vi "main.vi"() -> ()   [LabVIEW 2023]
panel:
  out "6-5 2":string
  out "6-4 2":string
  out "6-3 2":string
  out "6-2 2":string
  out "6-1 2":string
  out "5-5 2":string
  out "5-4 2":string
  out "5-3 2":string
  out "5-2 2":string
  out "5-1 2":string
  out "4-5 2":string
  out "4-4 2":string
  out "4-3 2":string
  out "4-2 2":string
  out "4-1 2":string
  out "3-5 2":string
  out "3-4 2":string
  out "3-3 2":string
  out "3-2 2":string
  out "3-1 2":string
  out "2-5 2":string
  out "2-4 2":string
  out "2-3 2":string
  out "2-2 2":string
  out "2-1 2":string
  out "1-5 2":string
  out "1-4 2":string
  out "1-3 2":string
  out "1-2 2":string
  out "1-1 2":string
  out "Class Name":string
  out "row":i32
  out "column":i32
  in  "BACKSPACE":bool
  in  "M":bool
  in  "N":bool
  in  "B":bool
  in  "V":bool
  in  "C":bool
  in  "X":bool
  in  "Z":bool
  in  "ENTER":bool
  in  "L":bool
  in  "K":bool
  in  "J":bool
  in  "H":bool
  in  "G":bool
  in  "F":bool
  in  "D":bool
  in  "S":bool
  in  "A":bool
  in  "P":bool
  in  "O":bool
  in  "I":bool
  in  "U":bool
  in  "Y":bool
  in  "T":bool
  in  "R":bool
  in  "E":bool
  in  "W":bool
  in  "Q":bool
  out "6-5":string
  out "6-4":string
  out "6-3":string
  out "6-2":string
  out "6-1":string
  out "5-5":string
  out "5-4":string
  out "5-3":string
  out "5-2":string
  out "5-1":string
  out "4-5":string
  out "4-4":string
  out "4-3":string
  out "4-2":string
  out "4-1":string
  out "3-5":string
  out "3-4":string
  out "3-3":string
  out "3-2":string
  out "3-1":string
  out "2-5":string
  out "2-4":string
  out "2-3":string
  out "2-2":string
  out "2-1":string
  out "1-5":string
  out "1-4":string
  out "1-3":string
  out "1-2":string
  out "1-1":string
  out "Array 2":string[](array[string])
  out "Array 3":string[][](array[string])
  # "Wordle"
  # "Wordle AI"
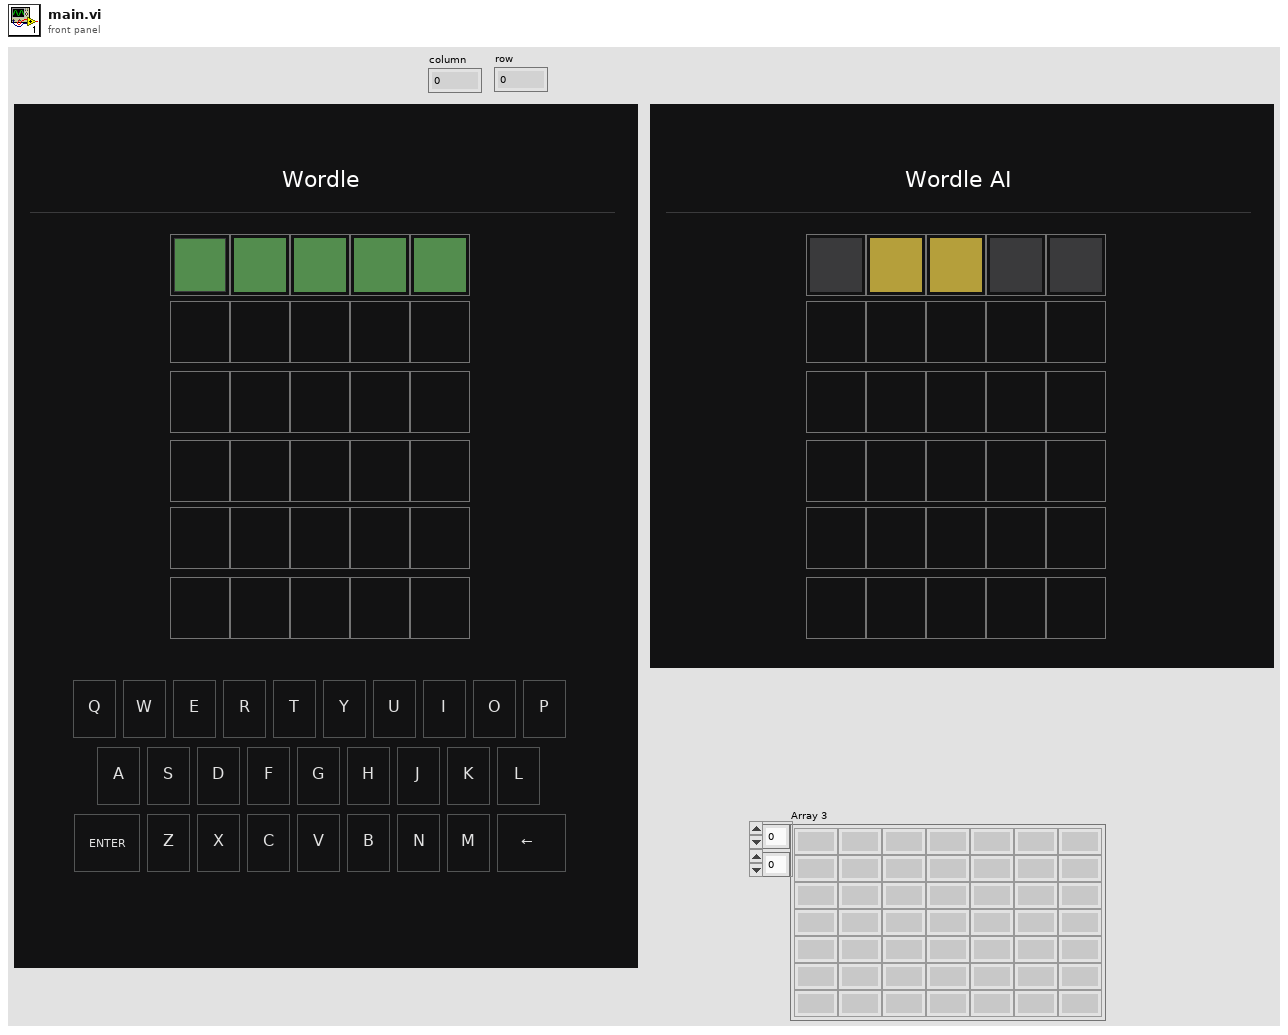
[diagram p1: front panel]
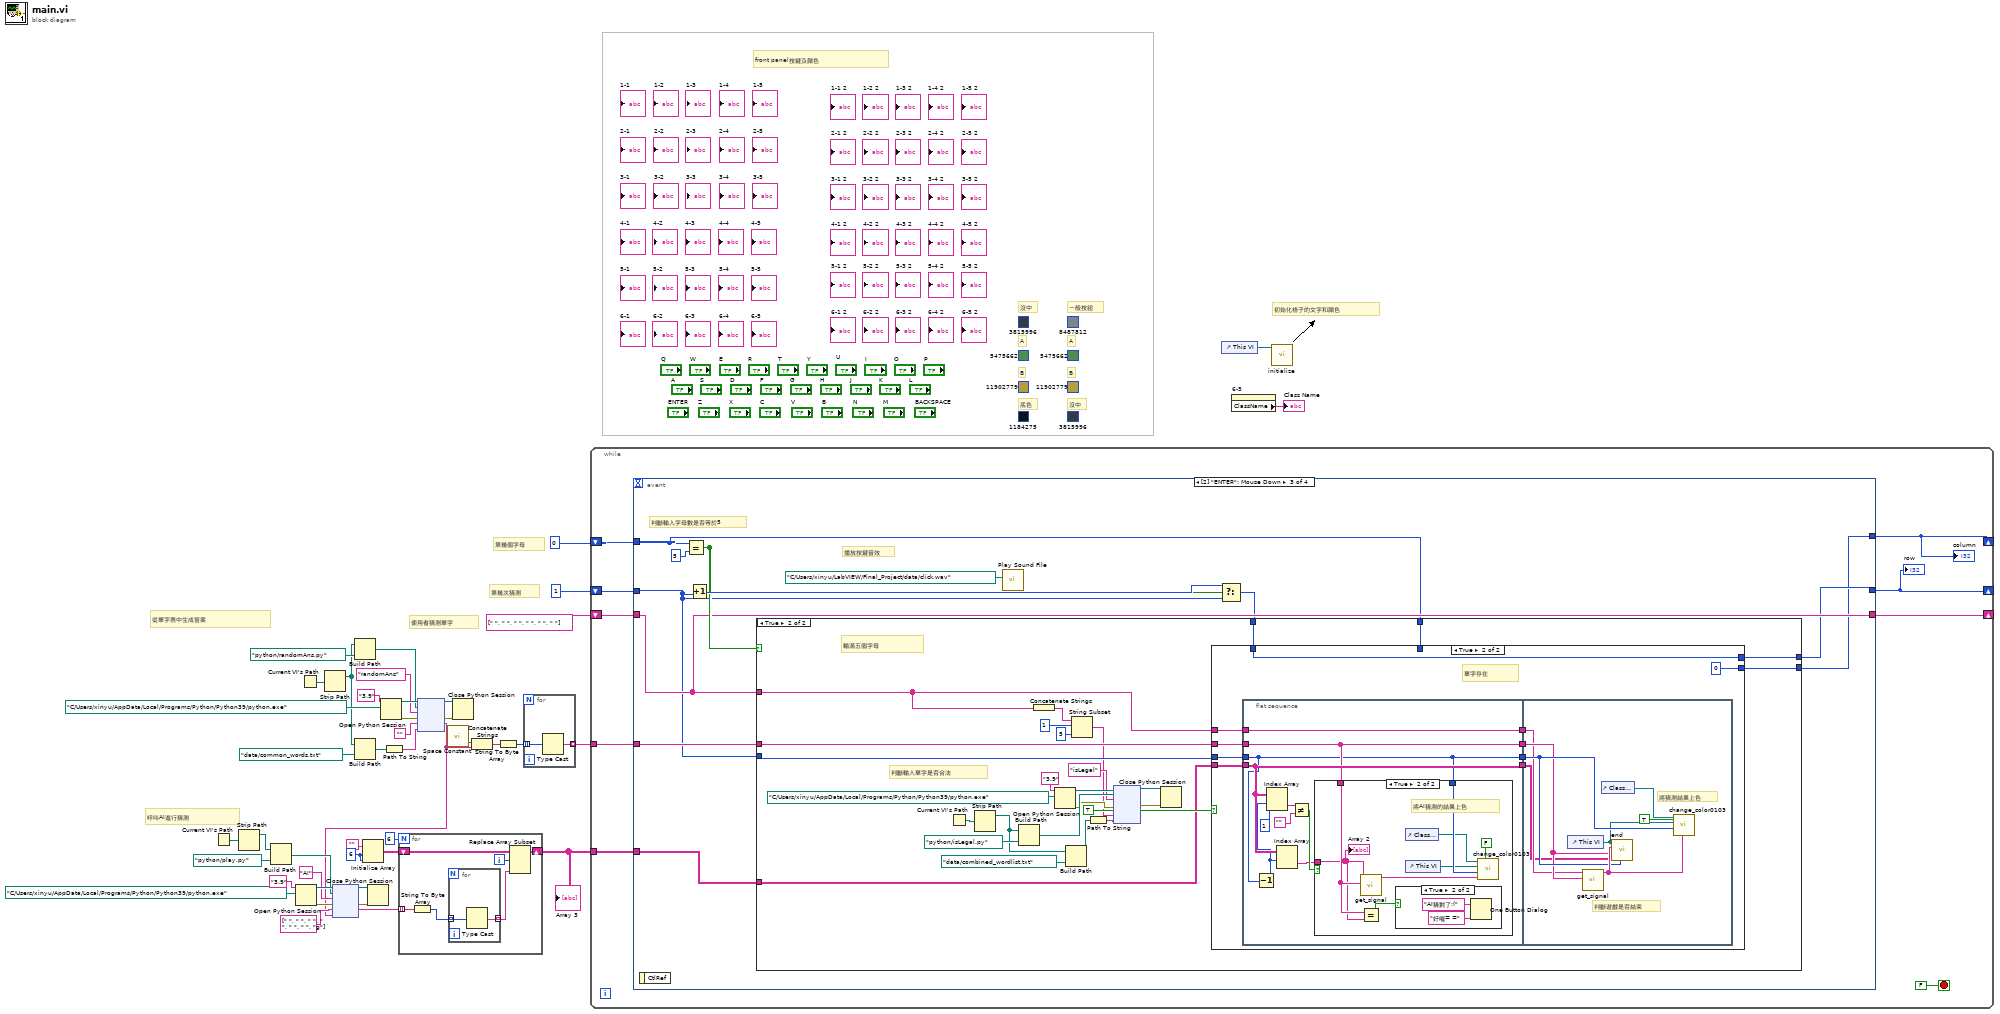
[diagram p0: block diagram]
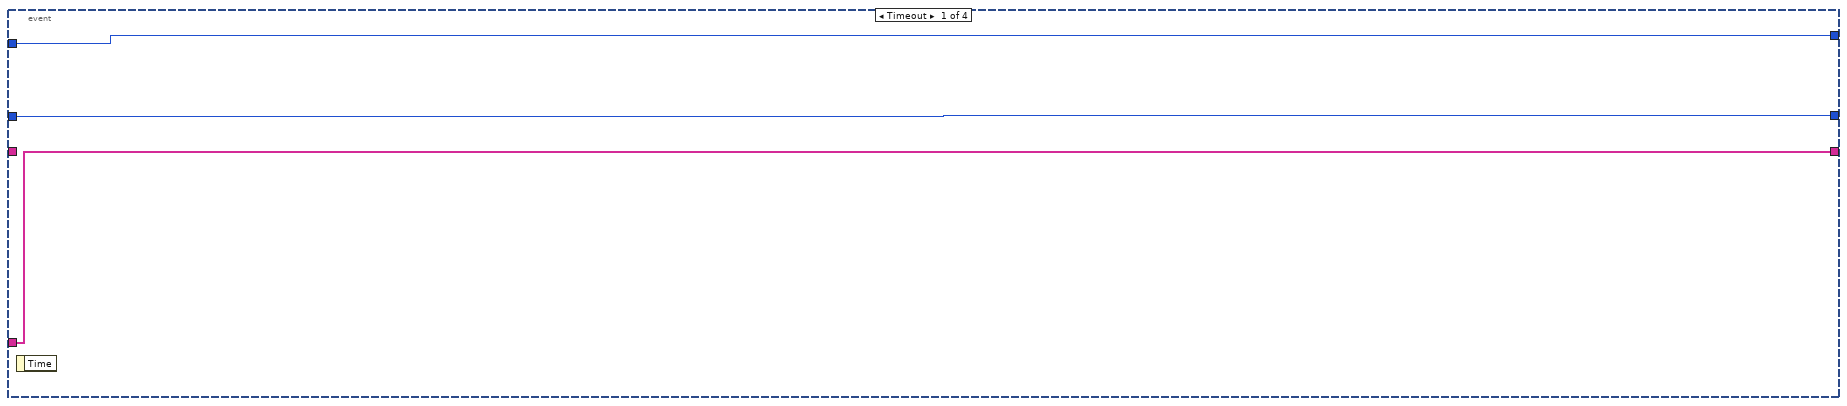
[diagram p2: hidden frame]
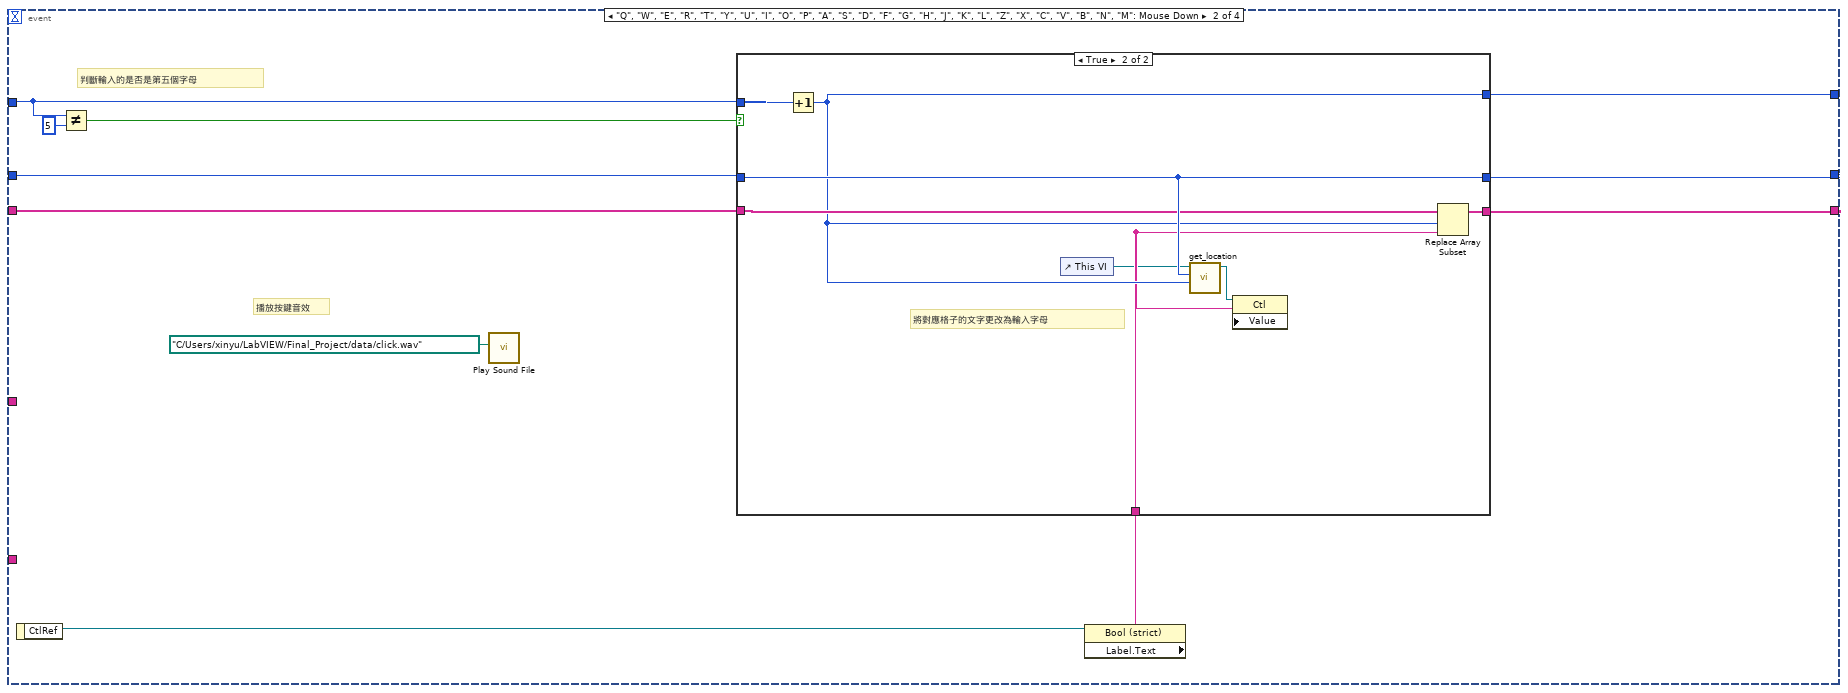
[diagram p3: hidden frame]
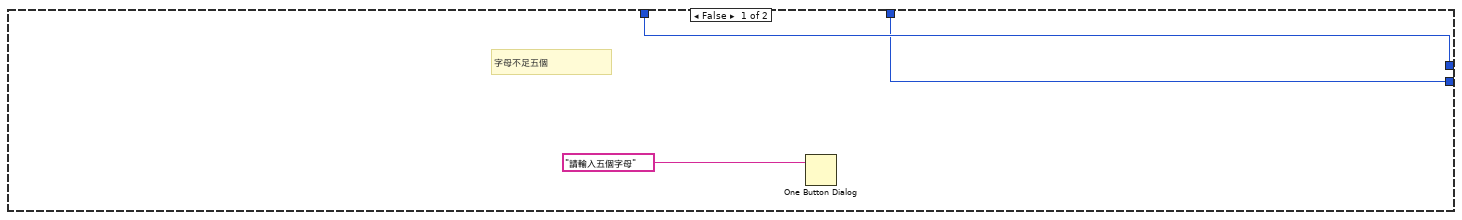
[diagram p5: hidden frame]
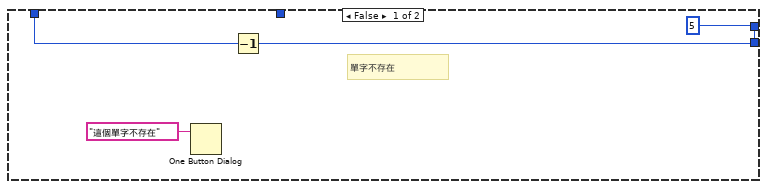
[diagram p6: hidden frame]
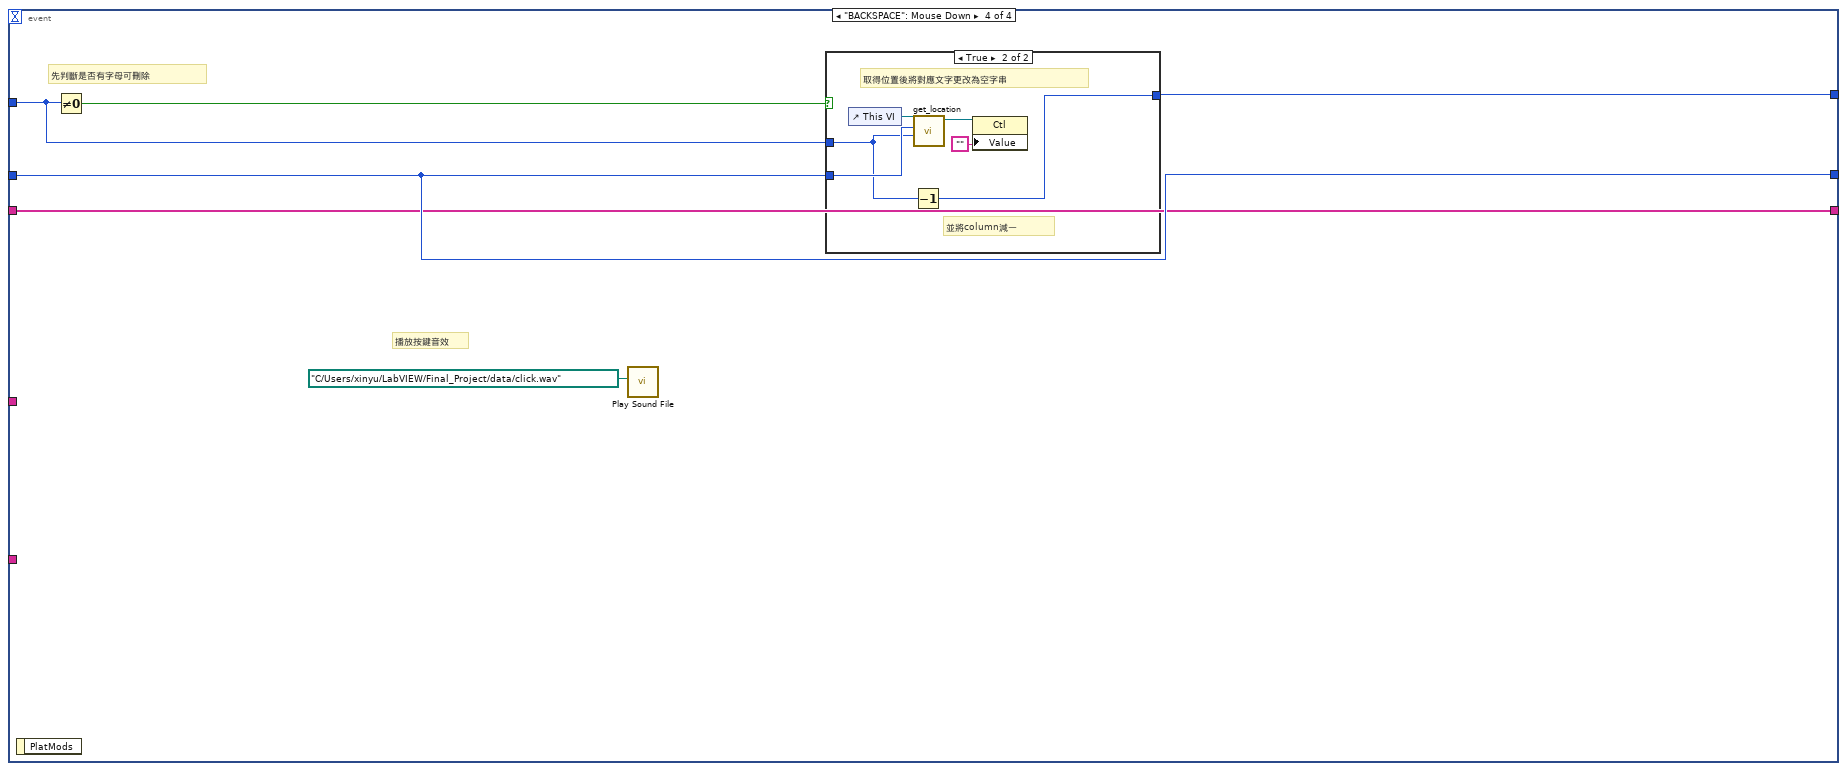
[diagram p9: hidden frame]
diagram:
  w1 = 6 ("dimension size")
  (unwired) u32 11902779 ("Text.Text Colors:BG Color")
  (unwired) u32 5475662 ("Text.Text Colors:BG Color")
  (unwired) u32 8487812 ("Text.Text Colors:BG Color")
  (unwired) u32 3815996 ("Text.Text Colors:BG Color")
  (unwired) u32 11902779 ("Text.Text Colors:BG Color")
  (unwired) u32 5475662 ("Text.Text Colors:BG Color")
  (unwired) u32 3815996 ("Text.Text Colors:BG Color")
  (unwired) u32 1184275 ("Text.Text Colors:BG Color")
  # "呼叫AI進行猜測"
  # "從單字表中生成答案"
  # "使用者猜測單字"
  # "初始化格子的文字和顏色"
  # "front panel按鍵及顏色"
  # "第幾次猜測"
  # "第幾個字母"
  # "沒中"
  # "B"
  # "A"
  # "一般按鈕"
  # "底色"
  # "B"
  # "A"
  # "沒中"
  n1 = Current VI's Path() -> (path=w17:path)
  n2 = Strip Path(path=w17) -> (stripped path=w14:path)  [unwired: 1 out]
  n3 = Build Path(base path=w14, name or relative path=path "python/play.py") -> (appended path=w11:path)
  n4 = Open Python Session(python version="3.9" ("Python version"), python path=path "C:/Users/xinyu/AppData/Local/Programs/Python/Python39/python.exe" ("Python path")) -> (session out=w16:refnum<k35>, error out=w15:errorcluster)  [unwired: 1 in]
  n5 = Current VI's Path() -> (path=w33:path)
  n6 = Strip Path(path=w33) -> (stripped path=w29:path)  [unwired: 1 out]
  n7 = Build Path(base path=w29, name or relative path=path "python/randomAns.py") -> (appended path=w24:path)
  n8 = Build Path(base path=w29, name or relative path=path "data/common_words.txt") -> (appended path=w36:path)
  n9 = Initialize Array("", w1, w1) -> (w10:string[][])
  n10 = Open Python Session(python version="3.9" ("Python version"), python path=path "C:/Users/xinyu/AppData/Local/Programs/Python/Python39/python.exe" ("Python path")) -> (session out=w32:refnum<k35>, error out=w31:errorcluster)  [unwired: 1 in]
  n11 = Path To String(path=w36) -> (string=w27:string)
  n12 = node(w32, w24, "randomAns" ("function name"), w31, "", w27) -> (w26:refnum<k35>, w25:errorcluster, w3:string)  [unwired: 1 in, 2 out]
  n13 = node(w16, w11, "AI" ("function name"), w15, string[] [" ", " ", " ", " ", " ", " ", "g"], w3) -> (w13:refnum<k35>, w12:errorcluster, w5:string[])  [unwired: 1 in, 2 out]
  n14 = Close Python Session(session in=w13, error in=w12) -> ()  [unwired: 1 out]
  n15 = for {
    N: 6 -> [_]
    shift-right: [w46] -> w4
    shift-left: w10 -> [w49]
    tunnel: w5 -> [w44] mode=indexing
    i -> [w47]
    n16 = String To Byte Array(string=w44) -> (unsigned byte array=w45:u8[])
    n17 = for {
      tunnel: w45 -> [w51] mode=indexing
      tunnel: [w50] -> w48 mode=indexing
      n18 = Type Cast(x=w51) -> (*(type *) &x=w50:string)  [unwired: 1 in]
    }
    n19 = Replace Array Subset(array=w49, new element=w48, index (row)=w47) -> (w46:string[][])  [unwired: 1 in]
  }
  "Array 3" <- w4
  n20 = call <vilib>:"Space Constant.vi"() -> ("String"=w23:string)
  n21 = Close Python Session(session in=w26, error in=w25) -> ()  [unwired: 1 out]
  n22 = Concatenate Strings(w23, w3) -> (w22:string)
  n23 = String To Byte Array(string=w22) -> (unsigned byte array=w21:u8[])
  n24 = for {
    tunnel: w21 -> [w53] mode=indexing
    tunnel: [w52] -> w2 mode=indexing
    n25 = Type Cast(x=w53) -> (*(type *) &x=w52:string)  [unwired: 1 in]
  }
  n26 = while {
    shift-right: [w60] -> _
    shift-left: 0 -> [w61]
    shift-right: [w54] -> _
    shift-left: 1 -> [w59]
    shift-right: [w58] -> _
    shift-left: string[] [" ", " ", " ", " ", " ", " "] -> [w55]
    tunnel: w2 -> [w57]
    tunnel: w4 -> [w56]
    stop <- FALSE stop-if-true
    n27 = event shown="[2] \"ENTER\": Mouse Down" {
      selector: _ -> [_ _ _ _]
      dyn-events: _ -> [_ _ _ _]
      timeout: _ -> [_ _ _ _]
      tunnel: w61 -> [w65 w73 w90 w177]
      tunnel: [w65 w72 w91 w176] -> w60
      tunnel: w59 -> [w64 w71 w94 w175]
      tunnel: [w64 w70 w92 w175] -> w54
      tunnel: w55 -> [_ w68 w95 w174]
      tunnel: [w63 w67 w95 w174] -> w58
      tunnel: w57 -> [w63 _ w96 _]
      tunnel: w56 -> [_ _ w89 _]
      event Timeout {
        n28 = event-data() -> ()  [unwired: 1 in, 1 out]
      }
      event "Q", "W", "E", "R", "T", "Y", "U", "I", "O", "P", "A", "S", "D", "F", "G", "H", "J", "K", "L", "Z", "X", "C", "V", "B", "N", "M": Mouse Down {
        # "播放按鍵音效"
        # "判斷輸入的是否是第五個字母"
        n29 = event-data() -> ("CtlRef"=w76:refnum<vi>)  [unwired: 1 in]
        n30 = Not Equal?(x=w73, y=5) -> (x != y?=w74:bool)
        n31 = call <vilib>:"Play Sound File.vi"("path"=path "C:/Users/xinyu/LabVIEW/Final_Project/data/click.wav") -> ()  [unwired: 9 in, 2 out]
        n32 = property class="Bool (strict)"(reference=w76) -> ("Label.Text"=w69:string)  [unwired: 1 in, 2 out]
        n33 = case shown="True" w74 {
          tunnel: w73 -> [w79 w87]
          tunnel: [w79 w83] -> w72
          tunnel: w71 -> [w78 w86]
          tunnel: [w78 w86] -> w70
          tunnel: w69 -> [_ w82]
          tunnel: w68 -> [w77 w84]
          tunnel: [w77 w81] -> w67
          frame False {
          }
          frame True {
            # "將對應格子的文字更改為輸入字母"
            n34 = Increment(x=w87) -> (x+1=w83:i32)
            n35 = control-ref of="This VI"() -> (w80:refnum<vi>)
            n36 = call "get_location.vi"("column"=w83, "row"=w86, "vi ref"=w80) -> ("letter ref"=w85:refnum<vi>)  [unwired: 8 in]
            n37 = property class="Ctl"(reference=w85, "Value"=w82) -> ()  [unwired: 1 in, 2 out]
            n38 = Replace Array Subset(array=w84, new element=w82, index=w83) -> (w81:string[])
          }
        }
      }
      event "ENTER": Mouse Down {
        # "播放按鍵音效"
        # "判斷輸入字母數是否等於5"
        n39 = event-data() -> ()  [unwired: 1 in, 1 out]
        n40 = Equal?(x=w90, y=5) -> (x = y?=w97:bool)
        n41 = Increment(x=w94) -> (x+1=w98:i32)
        n42 = call <vilib>:"Play Sound File.vi"("path"=path "C:/Users/xinyu/LabVIEW/Final_Project/data/click.wav") -> ()  [unwired: 9 in, 2 out]
        n43 = Select(t=w98, s=w97, f=w94) -> (s? t:f=w93:i32)
        n44 = case shown="True" w97 {
          tunnel: w95 -> [_ w114]
          tunnel: w96 -> [_ w130]
          tunnel: w94 -> [_ w129]
          tunnel: w93 -> [w101 w107]
          tunnel: [w101 w106] -> w92
          tunnel: [w100 w105] -> w91
          tunnel: w90 -> [w100 w104]
          tunnel: w89 -> [_ w103]
          frame False {
            # "字母不足五個"
            n45 = One Button Dialog(message="請輸入五個字母") -> ()  [unwired: 1 in, 1 out]
          }
          frame True {
            # "判斷輸入單字是否合法"
            # "輸滿五個字母"
            n46 = Current VI's Path() -> (path=w127:path)
            n47 = Strip Path(path=w127) -> (stripped path=w122:path)  [unwired: 1 out]
            n48 = Build Path(base path=w122, name or relative path=path "python/isLegal.py") -> (appended path=w124:path)
            n49 = Concatenate Strings(w114) -> (w110:string)
            n50 = Open Python Session(python version="3.9" ("Python version"), python path=path "C:/Users/xinyu/AppData/Local/Programs/Python/Python39/python.exe" ("Python path")) -> (session out=w125:refnum<k35>, error out=w118:errorcluster)  [unwired: 1 in]
            n51 = Build Path(base path=w122, name or relative path=path "data/combined_wordlist.txt") -> (appended path=w116:path)
            n52 = String Subset(string=w110, offset (0)=1, length (rest)=5 ("length (rest)")) -> (substring=w108:string)
            n53 = Path To String(path=w116) -> (string=w115:string)
            n54 = node(w125, w124, "isLegal" ("function name"), w118, TRUE, w108, w115) -> (w120:refnum<k35>, w119:errorcluster, w112:bool)  [unwired: 2 in, 2 out]
            n55 = Close Python Session(session in=w120, error in=w119) -> ()  [unwired: 1 out]
            n56 = case shown="True" w112 {
              tunnel: w114 -> [_ w141]
              tunnel: w130 -> [_ w137]
              tunnel: w129 -> [_ w135]
              tunnel: w107 -> [w133 w144]
              tunnel: [w132 w144] -> w106
              tunnel: [5 0] -> w105
              tunnel: w104 -> [_ _]
              tunnel: w103 -> [_ w139]
              frame False {
                # "單字不存在"
                n57 = One Button Dialog(message="這個單字不存在") -> ()  [unwired: 1 in, 1 out]
                n58 = Decrement(x=w133) -> (x-1=w132:i32)
              }
              frame True {
                # "單字存在"
                n59 = flat-sequence {
                  tunnel: w135 -> [w146]
                  tunnel: w139 -> [w148]
                  tunnel: w137 -> [w147]
                  tunnel: [w149] -> w142
                  tunnel: w141 -> [w149]
                  tunnel: [w148] -> w140
                  tunnel: [w147] -> w138
                  tunnel: [w146] -> w136
                  tunnel: w142 -> [w167]
                  tunnel: w140 -> [w166]
                  tunnel: w138 -> [w168]
                  tunnel: w136 -> [w169]
                  frame #0 {
                    n60 = Decrement(x=w146) -> (x-1=w145:i32)
                    n61 = Index Array(array=w148, index (row)=w145, index (col)=1 ("disabled index (col)")) -> (element=w153:string)
                    n62 = Index Array(array=w148, index (row)=w145) -> (element=w150:string[])  [unwired: 1 in]
                    n63 = Not Equal?(x=w153, y="") -> (x != y?=w151:bool)
                    n64 = case shown="True" w151 {
                      tunnel: w147 -> [_ w157]
                      tunnel: w150 -> [_ w156]
                      tunnel: w146 -> [_ w162]
                      frame False {
                      }
                      frame True {
                        # "將AI猜測的結果上色"
                        n65 = call "get_signal.vi"("Answer"=w157, "Guess"=w156) -> ("Signal"=w158:string[])  [unwired: 9 in]
                        n66 = Equal?(x=w157, y=w156) -> (x = y?=w155:bool)
                        n67 = case shown="True" w155 {
                          frame False {
                          }
                          frame True {
                            n68 = One Button Dialog(message="AI猜對了:(", button name ("OK")="好喔= =") -> ()  [unwired: 1 out]
                          }
                        }
                        n69 = control-ref of="Class Name"() -> (w160:refnum<vi>)
                        n70 = control-ref of="This VI"() -> (w161:refnum<vi>)
                        n71 = call "change_color0103.vi"("Signal"=w158, "isHuman"=FALSE, "row"=w162, "VI"=w161, "ref in"=w160) -> ()  [unwired: 7 in]
                        "Array 2" <- w156
                      }
                    }
                  }
                  frame #1 {
                    # "將猜測結果上色"
                    # "判斷遊戲是否結束"
                    n72 = control-ref of="This VI"() -> (w165:refnum<vi>)
                    n73 = call "get_signal.vi"("Answer"=w168, "Guess"=w167) -> ("Signal"=w172:string[])  [unwired: 9 in]
                    n74 = control-ref of="Class Name"() -> (w171:refnum<vi>)
                    n75 = call "end.vi"("row"=w169, "AI guess"=w166, "answer"=w168, "signal"=w172, "VI in"=w165) -> ()  [unwired: 7 in]
                    n76 = call "change_color0103.vi"("Signal"=w172, "isHuman"=TRUE ("s"), "row"=w169, "VI"=w165, "ref in"=w171) -> ()  [unwired: 7 in]
                  }
                }
              }
            }
          }
        }
      }
      event "BACKSPACE": Mouse Down {
        # "播放按鍵音效"
        # "先判斷是否有字母可刪除"
        n77 = event-data() -> ()  [unwired: 1 in, 1 out]
        n78 = Not Equal To 0?(x=w177) -> (x != 0?=w178:bool)
        n79 = call <vilib>:"Play Sound File.vi"("path"=path "C:/Users/xinyu/LabVIEW/Final_Project/data/click.wav") -> ()  [unwired: 9 in, 2 out]
        n80 = case shown="True" w178 {
          tunnel: w175 -> [_ w185]
          tunnel: w177 -> [w179 w181]
          tunnel: [w179 w180] -> w176
          frame False {
            # "沒有字母可刪除的話\ncolumn保持原樣"
          }
          frame True {
            # "並將column減一"
            # "取得位置後將對應文字更改為空字串"
            n81 = control-ref of="This VI"() -> (w184:refnum<vi>)
            n82 = Decrement(x=w181) -> (x-1=w180:i32)
            n83 = call "get_location.vi"("column"=w181, "row"=w185, "vi ref"=w184) -> ("letter ref"=w183:refnum<vi>)  [unwired: 8 in]
            n84 = property class="Ctl"(reference=w183, "Value"="") -> ()  [unwired: 1 in, 2 out]
          }
        }
      }
    }
    "column" <- w60
    "row" <- w54
  }
  n85 = control-ref of="This VI"() -> (w39:refnum<vi>)
  n86 = property on="6-5" class="Str"() -> ("ClassName"=→"Class Name":string)  [unwired: 2 in, 2 out]
  n87 = call "initialize.vi"("VI in"=w39) -> ()  [unwired: 11 in]
